vi "Scripting_FindObjectsOnDiagram.vi"(0 "ViRef(Ignored If Not Wired)":refnum<vi>, 1 "NodeTypesToSearchFor":string[](array[string]), 2 "Diagram(Ignored If Not Wired)":refnum<vi>, 3 "Don'tSearchSubStructures(False)":bool, 5 "error in (no error)":errorcluster) -> (15 "Nodes":refnum<vi>[](array[refnum]), 19 "error out":errorcluster)   [LabVIEW 2012]
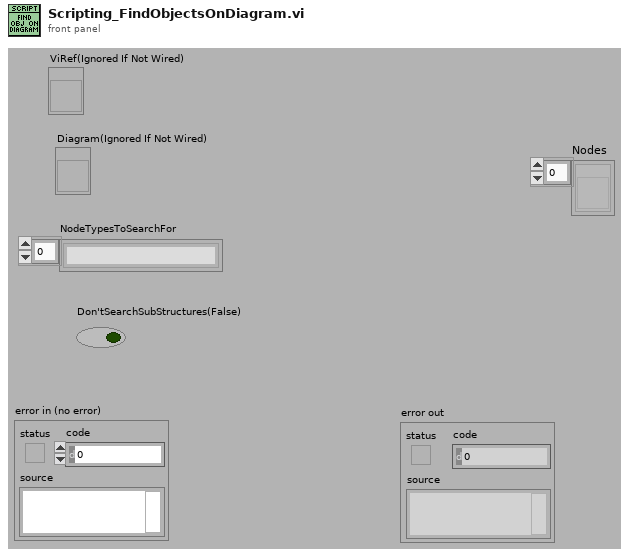
[diagram p1: front panel]
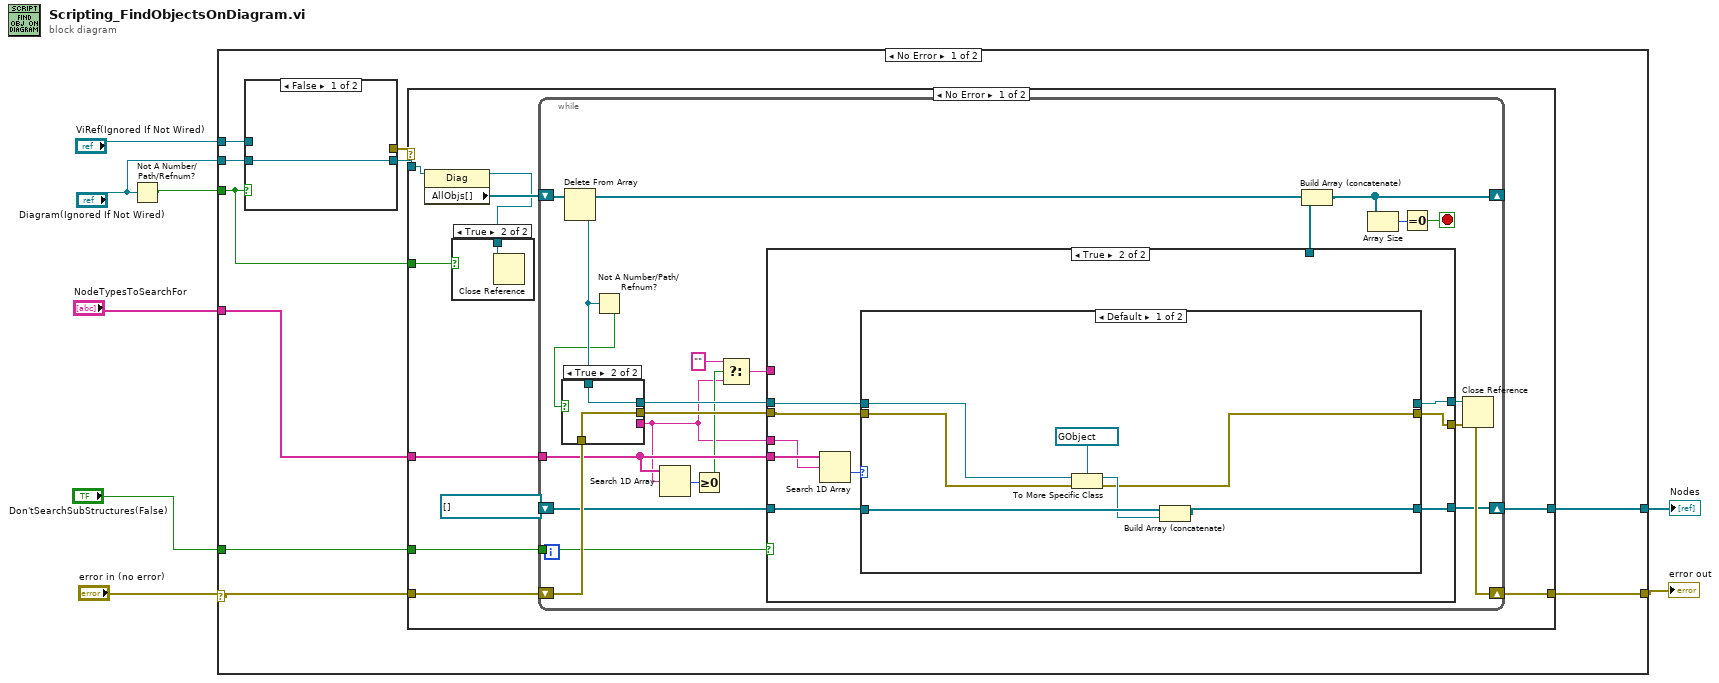
[diagram p0: block diagram]
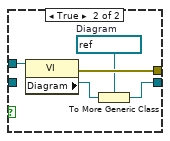
[diagram p2: hidden frame]
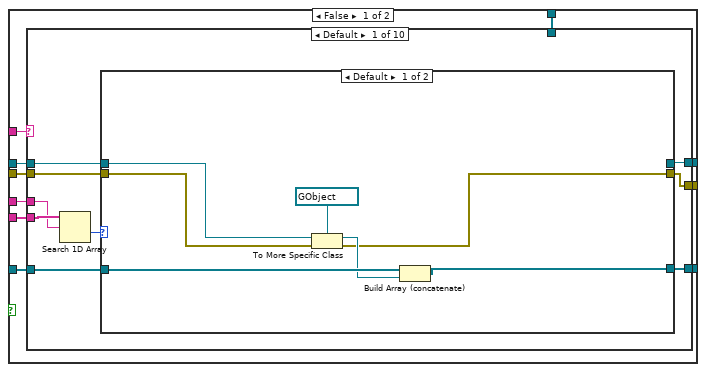
[diagram p4: hidden frame]
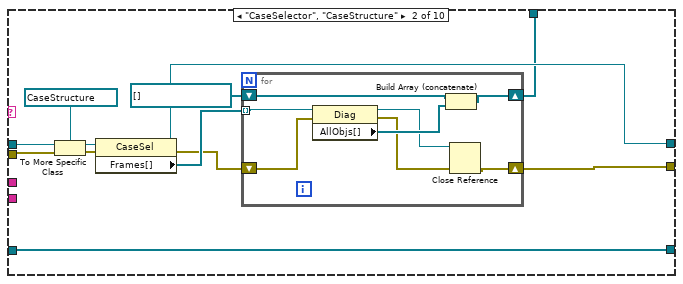
[diagram p6: hidden frame]
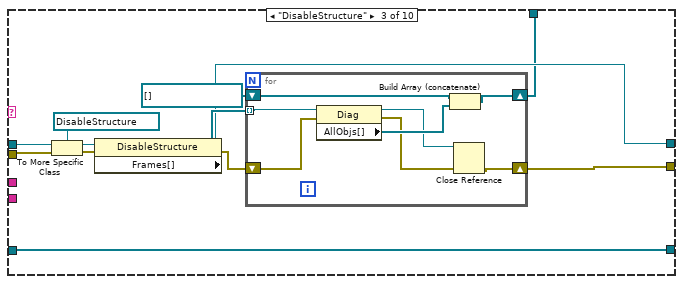
[diagram p7: hidden frame]
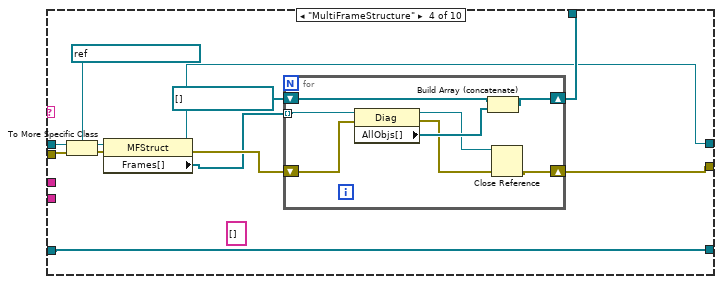
[diagram p8: hidden frame]
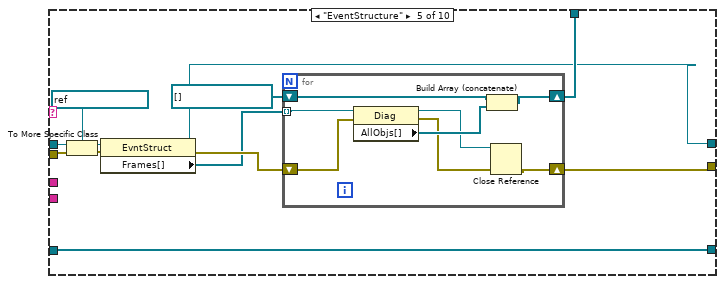
[diagram p9: hidden frame]
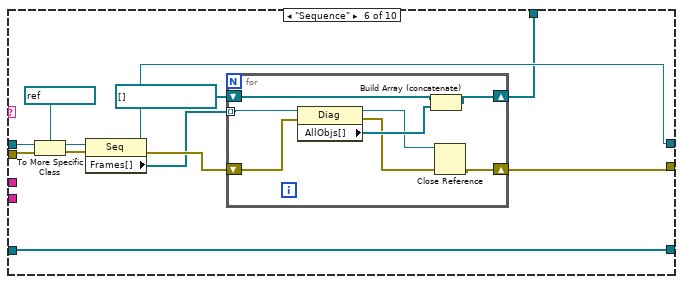
[diagram p10: hidden frame]
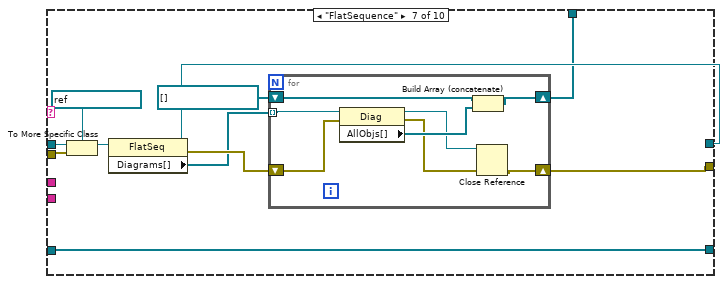
[diagram p11: hidden frame]
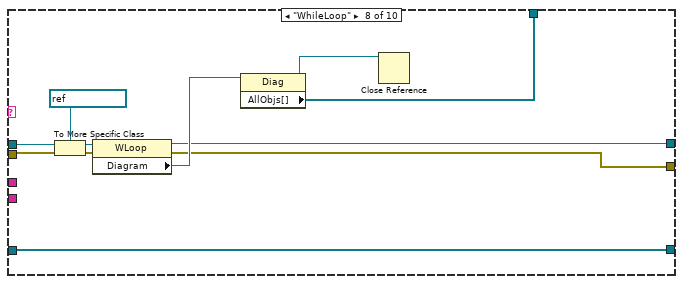
[diagram p12: hidden frame]
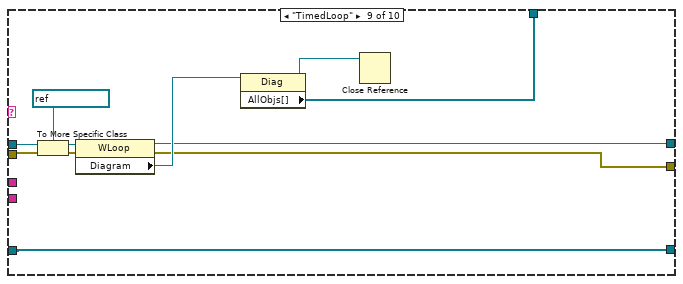
[diagram p13: hidden frame]
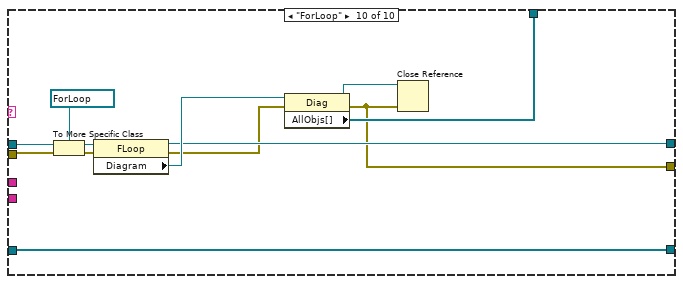
[diagram p14: hidden frame]
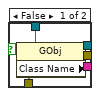
[diagram p16: hidden frame]
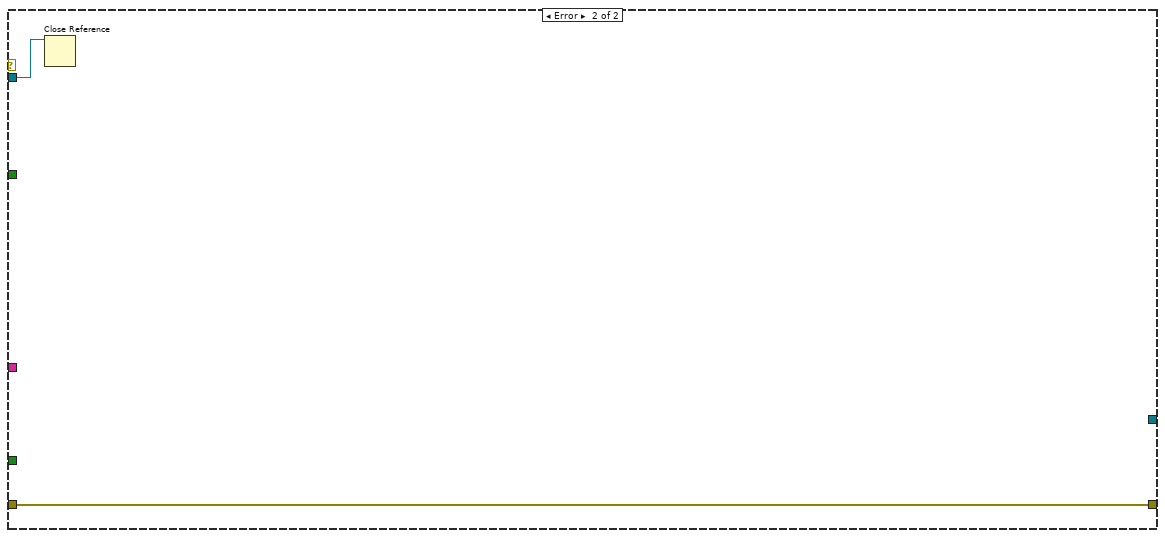
[diagram p17: hidden frame]
diagram:
  n1 = Not A Number/Path/Refnum?(number/path/refnum="Diagram(Ignored If Not Wired)") -> (NaN/Path/Refnum?=w3:bool)
  n2 = case shown="No Error" "error in (no error)" {
    selector: "error in (no error)" -> [w13 w268]
    tunnel: [w18 w268] -> w8
    tunnel: "NodeTypesToSearchFor" -> [w17 _]
    tunnel: "ViRef(Ignored If Not Wired)" -> [w16 _]
    tunnel: [w12 _] -> w4
    tunnel: w3 -> [w10 _]
    tunnel: "Diagram(Ignored If Not Wired)" -> [w11 _]
    tunnel: "Don'tSearchSubStructures(False)" -> [w9 _]
    frame No Error {
      n3 = case shown="False" w10 {
        tunnel: w16 -> [_ w24]
        tunnel: [w19 w20] -> w15
        tunnel: [_ w23] -> w14
        tunnel: w11 -> [w19 _]
        frame False {
        }
        frame True {
          w22 = refnum<vi> refnum  # Diagram
          n4 = property class="VI"(reference=w24) -> (error out=w23:errorcluster, "Diagram"=w21:refnum<vi>)  [unwired: 1 in, 1 out]
          n5 = To More Generic Class(target class=w22, reference=w21) -> (generic class reference=w20:refnum<vi>)
        }
      }
      n6 = case shown="No Error" w14 {
        tunnel: w15 -> [w34 w266]
        tunnel: [w32 w267] -> w18
        tunnel: w13 -> [w31 w267]
        tunnel: w17 -> [w30 _]
        tunnel: [w28 _] -> w12
        tunnel: w10 -> [w26 _]
        tunnel: w9 -> [w25 _]
        frame No Error {
          n7 = property class="Diag"(reference=w34) -> (reference out=w29:refnum<vi>, "AllObjs[]"=w33:refnum<vi>[])  [unwired: 1 in, 1 out]
          n8 = case shown="True" w26 {
            tunnel: w29 -> [_ w35]
            frame False {
            }
            frame True {
              n9 = Close Reference(reference=w35) -> ()  [unwired: 1 in, 1 out]
            }
          }
          n10 = while {
            shift-right: [w51] -> _
            shift-left: w33 -> [w57]
            shift-right: [w47] -> w32
            shift-left: w31 -> [w48]
            tunnel: w30 -> [w44]
            shift-right: [w45] -> w28
            shift-left: refnum<vi>[] [] ("Nodes") -> [w46]
            tunnel: w25 -> [w36]
            stop <- w55 stop-if-true
            n11 = Delete From Array(array=w57) -> (deleted portion=w38:refnum<vi>, array with subset deleted=w52:refnum<vi>[])  [unwired: 2 in]
            n12 = Not A Number/Path/Refnum?(number/path/refnum=w38) -> (NaN/Path/Refnum?=w37:bool)
            n13 = case shown="True" w37 {
              tunnel: [w263 w264] -> w54
              tunnel: [w262 w265] -> w53
              tunnel: w48 -> [w261 w264]
              tunnel: [w260 _] -> w41
              tunnel: w38 -> [w259 w265]
              frame False {
                n14 = property class="GObj"(reference=w259, error in=w261) -> (reference out=w262:refnum<vi>, error out=w263:errorcluster, "Class Name"=w260:string)
              }
              frame True {
              }
            }
            n15 = Search 1D Array(1D array=w44, element=w41) -> (index of element=w43:i32)  [unwired: 1 in]
            n16 = Greater Or Equal To 0?(x=w43) -> (x >= 0?=w42:bool)
            n17 = Select(t="", s=w42, f=w41) -> (s? t:f=w40:string)
            n18 = case shown="True" w36 {
              tunnel: w54 -> [w67 w243]
              tunnel: w53 -> [w66 w244]
              tunnel: [w65 _] -> w50
              tunnel: [w64 w246] -> w49
              tunnel: [w63 w245] -> w47
              tunnel: w46 -> [w62 w248]
              tunnel: [w61 w247] -> w45
              tunnel: w44 -> [w60 w242]
              tunnel: w41 -> [w59 w241]
              tunnel: w40 -> [w58 _]
              frame False {
                n19 = case shown="Default" w58 {
                  tunnel: w66 -> [w75 w98 w118 w138 w158 w178 w197 w216 w227 w239]
                  tunnel: w67 -> [w76 w93 w113 w135 w155 w175 w196 w212 w223 w235]
                  tunnel: [w73 w91 w111 w128 w149 w171 w189 w208 w219 w230] -> w63
                  tunnel: [_ w89 w109 w130 w150 w169 w188 w210 w221 w233] -> w65
                  tunnel: [w74 w92 w112 w129 w148 w170 w190 w209 w220 w232] -> w64
                  tunnel: w60 -> [w70 _ _ _ _ _ _ _ _ _]
                  tunnel: w62 -> [w72 w87 w107 w127 w147 w167 w187 w206 w217 w228]
                  tunnel: [w71 w87 w107 w127 w147 w167 w187 w206 w217 w228] -> w61
                  tunnel: w59 -> [w68 _ _ _ _ _ _ _ _ _]
                  frame Default {
                    n20 = Search 1D Array(1D array=w70, element=w68) -> (index of element=w69:i32)  [unwired: 1 in]
                    n21 = case shown="Default" w69 {
                      tunnel: w76 -> [w77 w86]
                      tunnel: w75 -> [w79 w85]
                      tunnel: [w78 w86] -> w73
                      tunnel: [_ w85] -> w74
                      tunnel: w72 -> [w83 w84]
                      tunnel: [w82 w84] -> w71
                      frame Default {
                        n22 = To More Specific Class(target class=refnum<vi> refnum ("WhileLoop"), reference=w79, error in=w77) -> (specific class reference=w81:refnum<vi>, error out=w78:errorcluster)
                        n23 = Build Array (concatenate)(w83, w81) -> (w82:refnum<vi>[])
                      }
                      frame -1 {
                      }
                    }
                  }
                  frame "CaseSelector", "CaseStructure" {
                    n24 = To More Specific Class(target class=refnum<vi> refnum ("CaseSelector"), reference=w98, error in=w93) -> (specific class reference=w96:refnum<vi>, error out=w94:errorcluster)
                    n25 = property class="CaseSel"(reference=w96, error in=w94) -> (reference out=w92:refnum<vi>, error out=w90:errorcluster, "Frames[]"=w95:refnum<vi>[])
                    n26 = for {
                      tunnel: w95 -> [w106] mode=indexing
                      shift-right: [w99] -> w91
                      shift-left: w90 -> [w105]
                      shift-right: [w102] -> w89
                      shift-left: refnum<vi>[] [] -> [w104]
                      n27 = property class="Diag"(reference=w106, error in=w105) -> (reference out=w100:refnum<vi>, error out=w101:errorcluster, "AllObjs[]"=w103:refnum<vi>[])
                      n28 = Build Array (concatenate)(w104, w103) -> (w102:refnum<vi>[])
                      n29 = Close Reference(reference=w100, error in (no error)=w101) -> (error out=w99:errorcluster)
                    }
                  }
                  frame "DisableStructure" {
                    n30 = To More Specific Class(target class=refnum<vi> refnum ("CaseSelector"), reference=w118, error in=w113) -> (specific class reference=w116:refnum<vi>, error out=w114:errorcluster)
                    n31 = property class="DisableStructure"(reference=w116, error in=w114) -> (reference out=w112:refnum<vi>, error out=w110:errorcluster, "Frames[]"=w115:refnum<vi>[])
                    n32 = for {
                      tunnel: w115 -> [w126] mode=indexing
                      shift-right: [w119] -> w111
                      shift-left: w110 -> [w125]
                      shift-right: [w122] -> w109
                      shift-left: refnum<vi>[] [] -> [w124]
                      n33 = property class="Diag"(reference=w126, error in=w125) -> (reference out=w120:refnum<vi>, error out=w121:errorcluster, "AllObjs[]"=w123:refnum<vi>[])
                      n34 = Build Array (concatenate)(w124, w123) -> (w122:refnum<vi>[])
                      n35 = Close Reference(reference=w120, error in (no error)=w121) -> (error out=w119:errorcluster)
                    }
                  }
                  frame "MultiFrameStructure" {
                    (unwired) string[] []
                    n36 = To More Specific Class(target class=refnum<vi> refnum ("MultiFrameStructure"), reference=w138, error in=w135) -> (specific class reference=w137:refnum<vi>, error out=w136:errorcluster)
                    n37 = property class="MFStruct"(reference=w137, error in=w136) -> (reference out=w129:refnum<vi>, error out=w132:errorcluster, "Frames[]"=w131:refnum<vi>[])
                    n38 = for {
                      tunnel: w131 -> [w146] mode=indexing
                      shift-right: [w139] -> w128
                      shift-left: w132 -> [w145]
                      shift-right: [w142] -> w130
                      shift-left: refnum<vi>[] [] -> [w144]
                      n39 = property class="Diag"(reference=w146, error in=w145) -> (reference out=w140:refnum<vi>, error out=w141:errorcluster, "AllObjs[]"=w143:refnum<vi>[])
                      n40 = Build Array (concatenate)(w144, w143) -> (w142:refnum<vi>[])
                      n41 = Close Reference(reference=w140, error in (no error)=w141) -> (error out=w139:errorcluster)
                    }
                  }
                  frame "EventStructure" {
                    n42 = To More Specific Class(target class=refnum<vi> refnum ("EventStructure"), reference=w158, error in=w155) -> (specific class reference=w157:refnum<vi>, error out=w156:errorcluster)
                    n43 = property class="EvntStruct"(reference=w157, error in=w156) -> (reference out=w148:refnum<vi>, error out=w152:errorcluster, "Frames[]"=w151:refnum<vi>[])
                    n44 = for {
                      tunnel: w151 -> [w166] mode=indexing
                      shift-right: [w159] -> w149
                      shift-left: w152 -> [w165]
                      shift-right: [w162] -> w150
                      shift-left: refnum<vi>[] [] -> [w164]
                      n45 = property class="Diag"(reference=w166, error in=w165) -> (reference out=w160:refnum<vi>, error out=w161:errorcluster, "AllObjs[]"=w163:refnum<vi>[])
                      n46 = Build Array (concatenate)(w164, w163) -> (w162:refnum<vi>[])
                      n47 = Close Reference(reference=w160, error in (no error)=w161) -> (error out=w159:errorcluster)
                    }
                  }
                  frame "Sequence" {
                    n48 = To More Specific Class(target class=refnum<vi> refnum ("Sequence"), reference=w178, error in=w175) -> (specific class reference=w177:refnum<vi>, error out=w176:errorcluster)
                    n49 = property class="Seq"(reference=w177, error in=w176) -> (reference out=w170:refnum<vi>, error out=w172:errorcluster, "Frames[]"=w168:refnum<vi>[])
                    n50 = for {
                      tunnel: w168 -> [w186] mode=indexing
                      shift-right: [w179] -> w171
                      shift-left: w172 -> [w185]
                      shift-right: [w182] -> w169
                      shift-left: refnum<vi>[] [] -> [w184]
                      n51 = property class="Diag"(reference=w186, error in=w185) -> (reference out=w180:refnum<vi>, error out=w181:errorcluster, "AllObjs[]"=w183:refnum<vi>[])
                      n52 = Build Array (concatenate)(w184, w183) -> (w182:refnum<vi>[])
                      n53 = Close Reference(reference=w180, error in (no error)=w181) -> (error out=w179:errorcluster)
                    }
                  }
                  frame "FlatSequence" {
                    n54 = To More Specific Class(target class=refnum<vi> refnum ("FlatSequence"), reference=w197, error in=w196) -> (specific class reference=w194:refnum<vi>)  [unwired: 1 out]
                    n55 = property class="FlatSeq"(reference=w194) -> (reference out=w190:refnum<vi>, error out=w192:errorcluster, "Diagrams[]"=w191:refnum<vi>[])  [unwired: 1 in]
                    n56 = for {
                      tunnel: w191 -> [w205] mode=indexing
                      shift-right: [w198] -> w189
                      shift-left: w192 -> [w204]
                      shift-right: [w201] -> w188
                      shift-left: refnum<vi>[] [] -> [w203]
                      n57 = property class="Diag"(reference=w205, error in=w204) -> (reference out=w199:refnum<vi>, error out=w200:errorcluster, "AllObjs[]"=w202:refnum<vi>[])
                      n58 = Build Array (concatenate)(w203, w202) -> (w201:refnum<vi>[])
                      n59 = Close Reference(reference=w199, error in (no error)=w200) -> (error out=w198:errorcluster)
                    }
                  }
                  frame "WhileLoop" {
                    n60 = To More Specific Class(target class=refnum<vi> refnum ("WhileLoop"), reference=w216, error in=w212) -> (specific class reference=w215:refnum<vi>, error out=w213:errorcluster)
                    n61 = property class="WLoop"(reference=w215, error in=w213) -> (reference out=w209:refnum<vi>, error out=w208:errorcluster, "Diagram"=w211:refnum<vi>)
                    n62 = property class="Diag"(reference=w211) -> (reference out=w207:refnum<vi>, "AllObjs[]"=w210:refnum<vi>[])  [unwired: 1 in, 1 out]
                    n63 = Close Reference(reference=w207) -> ()  [unwired: 1 in, 1 out]
                  }
                  frame "TimedLoop" {
                    n64 = To More Specific Class(target class=refnum<vi> refnum ("WhileLoop"), reference=w227, error in=w223) -> (specific class reference=w226:refnum<vi>, error out=w224:errorcluster)
                    n65 = property class="WLoop"(reference=w226, error in=w224) -> (reference out=w220:refnum<vi>, error out=w219:errorcluster, "Diagram"=w222:refnum<vi>)
                    n66 = property class="Diag"(reference=w222) -> (reference out=w218:refnum<vi>, "AllObjs[]"=w221:refnum<vi>[])  [unwired: 1 in, 1 out]
                    n67 = Close Reference(reference=w218) -> ()  [unwired: 1 in, 1 out]
                  }
                  frame "ForLoop" {
                    n68 = To More Specific Class(target class=refnum<vi> refnum ("WhileLoop"), reference=w239, error in=w235) -> (specific class reference=w238:refnum<vi>, error out=w236:errorcluster)
                    n69 = property class="FLoop"(reference=w238, error in=w236) -> (reference out=w232:refnum<vi>, error out=w231:errorcluster, "Diagram"=w234:refnum<vi>)
                    n70 = property class="Diag"(reference=w234, error in=w231) -> (reference out=w229:refnum<vi>, error out=w230:errorcluster, "AllObjs[]"=w233:refnum<vi>[])
                    n71 = Close Reference(reference=w229, error in (no error)=w230) -> ()  [unwired: 1 out]
                  }
                }
              }
              frame True {
                n72 = Search 1D Array(1D array=w242, element=w241) -> (index of element=w240:i32)  [unwired: 1 in]
                n73 = case shown="Default" w240 {
                  tunnel: w243 -> [w249 w258]
                  tunnel: w244 -> [w251 w257]
                  tunnel: [w250 w258] -> w245
                  tunnel: [_ w257] -> w246
                  tunnel: w248 -> [w255 w256]
                  tunnel: [w254 w256] -> w247
                  frame Default {
                    n74 = To More Specific Class(target class=refnum<vi> refnum ("WhileLoop"), reference=w251, error in=w249) -> (specific class reference=w253:refnum<vi>, error out=w250:errorcluster)
                    n75 = Build Array (concatenate)(w255, w253) -> (w254:refnum<vi>[])
                  }
                  frame -1 {
                  }
                }
              }
            }
            n76 = Build Array (concatenate)(w52, w50) -> (w51:refnum<vi>[])
            n77 = Array Size(array=w51) -> (size(s)=w56:i32)
            n78 = Equal To 0?(x=w56) -> (x = 0?=w55:bool)
            n79 = Close Reference(reference=w49, error in (no error)=w47) -> ()  [unwired: 1 out]
          }
        }
        frame Error {
          n80 = Close Reference(reference=w266) -> ()  [unwired: 1 in, 1 out]
        }
      }
    }
    frame Error {
    }
  }
  "error out" <- w8
  "Nodes" <- w4
